vi "Set Waveform Graph LegNumRows.vi"(4 "legend row holdoff":u32=1, 6 "legend row height":u32=23, 8 "error in":errorcluster, 11 "WaveformGraph":refnum<vi>) -> (0 "error out":errorcluster)   [LabVIEW 2018, in "NI_TDMS File Viewer.lvlib"]
uses:
  NI_TDMS File Viewer.lvlib
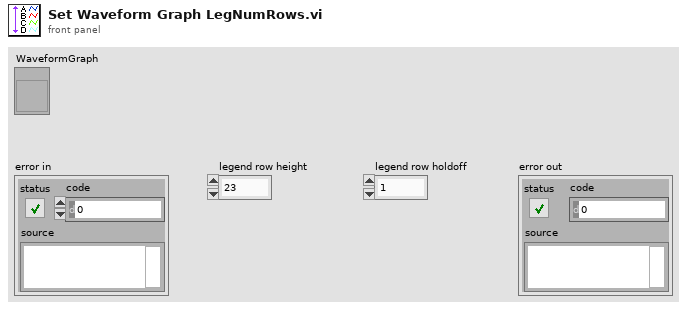
[diagram p1: front panel]
types:
  T1 = typedef "LVRectTypeDef.ctl" = cluster{"Left":i16, "Top":i16, "Right":i16, "Bottom":i16}
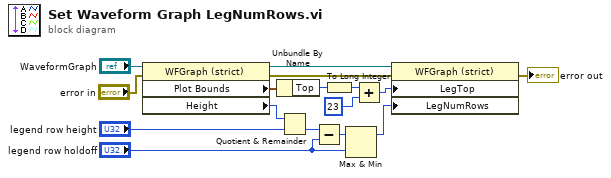
[diagram p0: block diagram]
diagram:
  n1 = property on="Property Node" class="WFGraph (strict)"(reference="WaveformGraph", error in="error in") -> (reference out=w9:refnum<vi>, error out=w14:errorcluster, "Plot Bounds"=w5:T1, "Height"=w6:u32)
  n2 = Unbundle By Name(w5) -> ("Top"=w4:i16)
  n3 = Quotient & Remainder(x=w6, y="legend row height") -> (floor(x/y)=w8:u32)  [unwired: 1 out]
  n4 = Subtract(x=w8, y="legend row holdoff") -> (x-y=w12:u32)
  n5 = To Long Integer(number=w4) -> (32bit integer=w1:i32)
  n6 = Max & Min(x=w12, y="legend row holdoff") -> (max(x,y)=w13:u32)  [unwired: 1 out]
  n7 = Add(x=w1, y=23) -> (x+y=w2:i32)
  n8 = property on="Property Node" class="WFGraph (strict)"(reference=w9, error in=w14, "LegTop"=w2, "LegNumRows"=w13) -> (error out=→"error out":errorcluster)  [unwired: 1 out]
